vi "标签查看.vi"(8 "error in":errorcluster caption="错误输入（无错误）", 11 "仓库路径":path=path "E:/学习文件/Git插件/test") -> (0 "error out":errorcluster caption="错误输出", 1 "standard error":string caption="标准错误", 2 "standard output":string[](array[string]) caption="标准输出", 3 "仓库路径":path=path "E:/学习文件/Git插件/test")   [LabVIEW 2018]
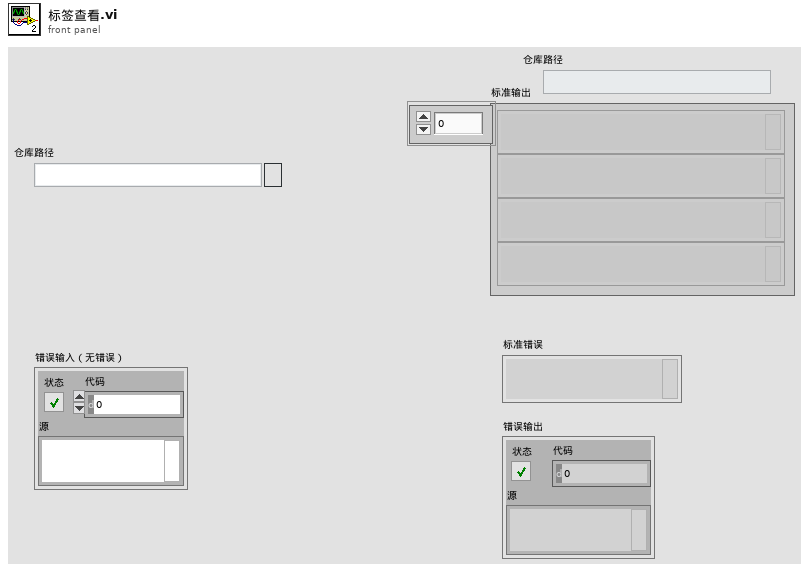
[diagram p1: front panel]
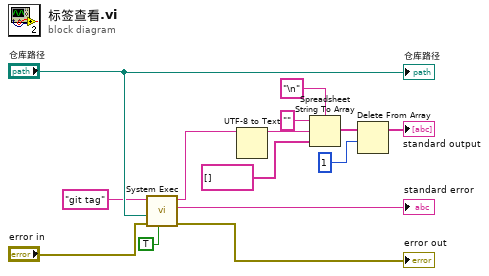
[diagram p0: block diagram]
diagram:
  n1 = call <vilib>:"System Exec.vi"("run minimized? (F)"=TRUE, "error in (no error)"="error in", "working directory"="仓库路径", "command line"="git tag") -> ("error out"=→"error out":errorcluster, "standard error"=→"standard error":string, "standard output"=w4:string)  [unwired: 4 in, 1 out]
  n2 = UTF-8 to Text ("UTF-8至文本转换")(11:w4) -> (3:w3:string)  [unwired: 2 in, 1 out]
  n3 = Spreadsheet String To Array(delimiter (Tab)="\n" ("分隔符(Tab)"), format string="" ("格式字符串"), spreadsheet string=w3, array type (2D Dbl)=string[] []) -> (array=w5:string[])
  n4 = Delete From Array(array=w5, length=1 ("长度")) -> (array with subset deleted=→"standard output":string[])  [unwired: 1 in, 1 out]
  "仓库路径" <- "仓库路径"
